vi "DetectCollisions.vi"(8 "error in (no error)":errorcluster, 9 "Collision Points":T1(array[cluster]), 10 "Position Delta":cluster{"X":sgl, "Y":sgl, "Z":sgl}, 11 "3D Scene in":refnum<class "3D Scene.lvclass">) -> (0 "error out":errorcluster, 2 "Adjusted Position Delta":cluster{"X":sgl, "Y":sgl, "Z":sgl}, 3 "3D Scene out":refnum<class "3D Scene.lvclass">)   [LabVIEW 2015, in "3D Scene.lvclass"]
uses:
  3D Scene.lvclass
  3D Scene.lvclass/3D Scene.ctl
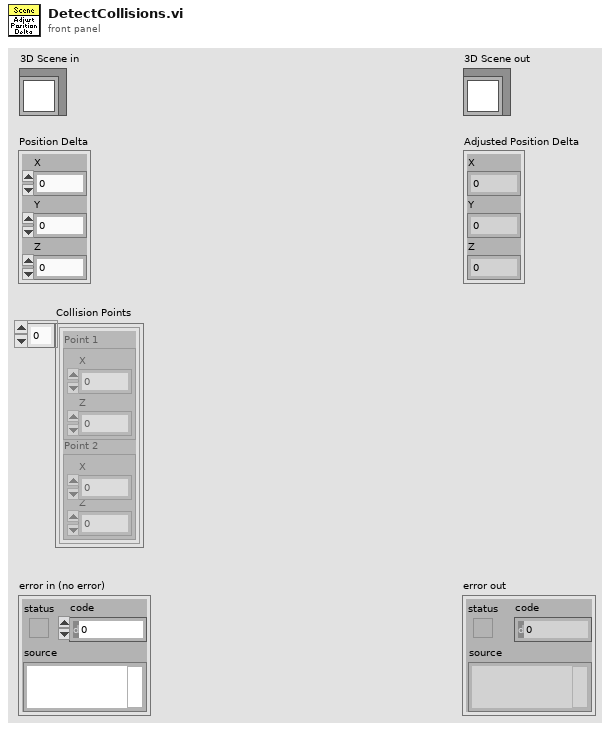
[diagram p1: front panel]
types:
  T1 = cluster{"Point 1":cluster{"Z":dbl, "X":dbl}, "Point 2":cluster{"Z":dbl, "X":dbl}}[]
  T2 = typedef "3D Point.ctl" = cluster{"X":sgl, "Y":sgl, "Z":sgl}
  T3 = cluster{cluster{"X":sgl, "Z":sgl}, cluster{sgl, "Z":sgl}}
  T4 = cluster{cluster{"X":sgl, "Z":sgl}, cluster{"X":sgl, sgl}}
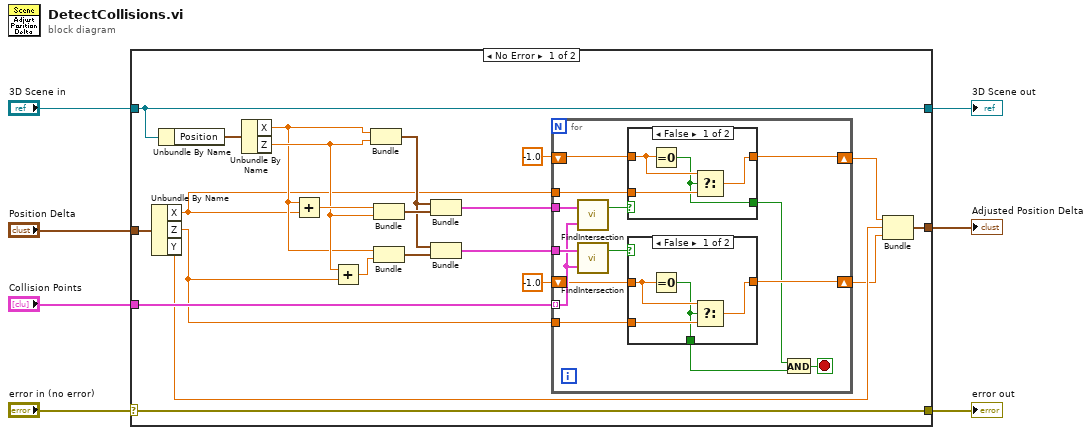
[diagram p0: block diagram]
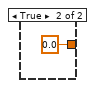
[diagram p2: hidden frame]
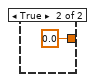
[diagram p3: hidden frame]
diagram:
  n1 = case shown="No Error" "error in (no error)" {
    selector: "error in (no error)" -> [w29 w55]
    tunnel: [w29 w55] -> w6
    tunnel: [w28 w54] -> w4
    tunnel: "3D Scene in" -> [w28 w54]
    tunnel: "Position Delta" -> [w25 _]
    tunnel: "Collision Points" -> [w26 _]
    tunnel: [w12 _] -> w1
    frame No Error {
      n2 = Unbundle By Name(w25) -> ("X"=w14:sgl, "Z"=w16:sgl, "Y"=w13:sgl)
      n3 = Unbundle By Name(w28) -> ("Position"=w24:T2)
      n4 = Unbundle By Name(w24) -> ("X"=w20:sgl, "Z"=w22:sgl)
      n5 = Add(x=w20, y=w14) -> (x+y=w23:sgl)
      n6 = Add(x=w22, y=w16) -> (x+y=w21:sgl)
      n7 = Bundle("X"=w20, "Z"=w22) -> (w18:cluster{"X":sgl, "Z":sgl})  [unwired: 1 in]
      n8 = Bundle(w23, "Z"=w22) -> (w27:cluster{sgl, "Z":sgl})  [unwired: 1 in]
      n9 = Bundle("X"=w20, w21) -> (w19:cluster{"X":sgl, sgl})  [unwired: 1 in]
      n10 = Bundle(w18, w27) -> (w15:T3)  [unwired: 1 in]
      n11 = Bundle(w18, w19) -> (w17:T4)  [unwired: 1 in]
      n12 = for {
        tunnel: w26 -> [w42] mode=indexing
        tunnel: w17 -> [w43]
        tunnel: w16 -> [w35]
        tunnel: w15 -> [w41]
        tunnel: w14 -> [w37]
        shift-right: [w38] -> w8
        shift-left: sgl -1.0 -> [w39]
        shift-right: [w33] -> w9
        shift-left: sgl -1.0 -> [w34]
        stop <- w32 stop-if-true
        n13 = call "FindIntersection.vi"("Segment B"=w42, "Segment A"=w41) -> ("Segments Intersect?"=w40:bool)  [unwired: 1 out]
        n14 = call "FindIntersection.vi"("Segment B"=w42, "Segment A"=w43) -> ("Segments Intersect?"=w36:bool)  [unwired: 1 out]
        n15 = case shown="False" w40 {
          tunnel: w39 -> [w52 _]
          tunnel: [w51 sgl 0.0] -> w38
          tunnel: w37 -> [w50 _]
          tunnel: [w49 _] -> w30
          frame False {
            n16 = Equal To 0?(x=w52) -> (x = 0?=w49:bool)
            n17 = Select(t=w52, s=w49, f=w50) -> (s? t:f=w51:sgl)
          }
          frame True {
          }
        }
        n18 = case shown="False" w36 {
          tunnel: [w47 sgl 0.0] -> w33
          tunnel: w35 -> [w46 _]
          tunnel: w34 -> [w45 _]
          tunnel: [w44 _] -> w31
          frame False {
            n19 = Equal To 0?(x=w45) -> (x = 0?=w44:bool)
            n20 = Select(t=w45, s=w44, f=w46) -> (s? t:f=w47:sgl)
          }
          frame True {
          }
        }
        n21 = And(x=w30, y=w31) -> (x .and. y?=w32:bool)
      }
      n22 = Bundle(w8, "Y"=w13, w9) -> (w12:cluster{sgl, "Y":sgl, sgl})  [unwired: 1 in]
    }
    frame Error {
    }
  }
  "error out" <- w6
  "3D Scene out" <- w4
  "Adjusted Position Delta" <- w1
